vi "assignment_cont.vi"() -> ()   [LabVIEW 2014]
uses:
  <vilib>/DAQmx/create/channels.llb/DAQmx Create Channel (AI-Voltage-Basic).vi
  <vilib>/DAQmx/read.llb/DAQmx Read (Analog 1D DBL NChan 1Samp).vi
  <vilib>/Utility/file.llb/Write To Spreadsheet File (string).vi
  <vilib>/Utility/file.llb/Write To Spreadsheet File (DBL).vi
panel:
  out "elapsed time(sec)":dbl
  out "XY Graph":cluster{dbl[], dbl[]}[](graph)
  in  "while loop delay time in sec":dbl
  in  "stop":bool
  in  "physical input channels":tag
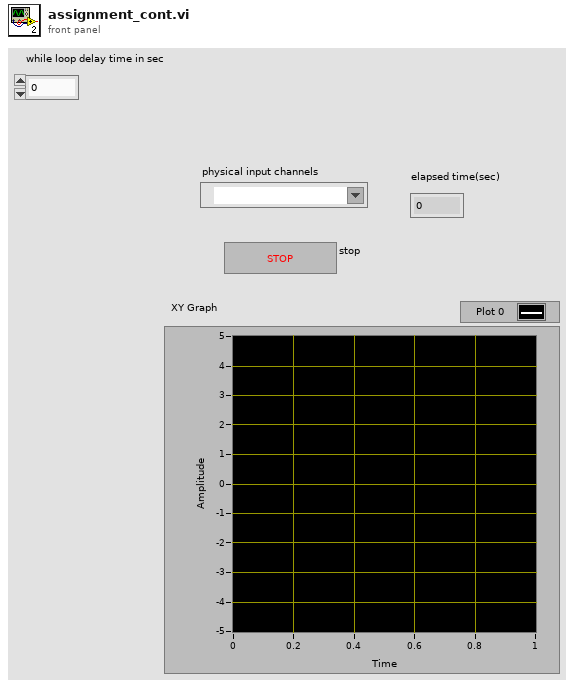
[diagram p1: front panel]
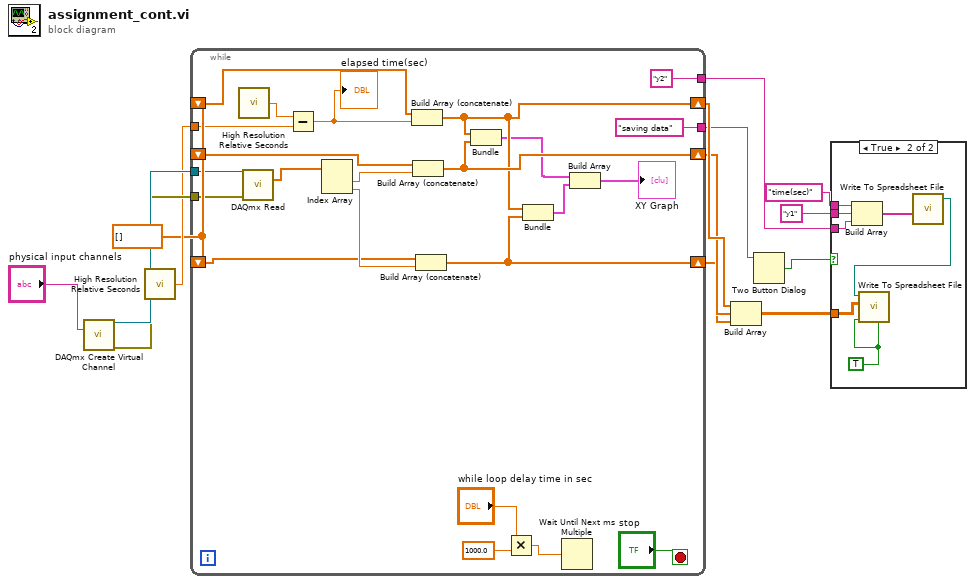
[diagram p0: block diagram]
diagram:
  w10 = dbl[] []
  n1 = call-poly <vilib>:"DAQmx Create Virtual Channel.vi"("physical channels"="physical input channels") -> ("task out"=w14:refnum<k21>, "error out"=w13:errorcluster)  [unwired: 13 in]
  n2 = call <vilib>:"High Resolution Relative Seconds.vi"() -> ("relative seconds"=w11:dbl)
  n3 = while {
    tunnel: w14 -> [w37]
    tunnel: w13 -> [w36]
    tunnel: w11 -> [w30]
    shift-right: [w22] -> w9
    shift-left: w10 -> [w29]
    shift-right: [w23] -> w8
    shift-left: w10 -> [w26]
    shift-right: [w21] -> w7
    shift-left: w10 -> [w24]
    tunnel: ["y2"] -> w3
    tunnel: ["saving data" ("message")] -> w1
    stop <- "stop" stop-if-true
    n4 = call <vilib>:"High Resolution Relative Seconds.vi"() -> ("relative seconds"=w31:dbl)
    n5 = call-poly <vilib>:"DAQmx Read.vi"("task/channels in"=w37, "error in"=w36) -> ("data"=w28:dbl[])  [unwired: 11 in, 2 out]
    n6 = Subtract(x=w31, y=w30) -> (x-y=w15:dbl)
    "elapsed time(sec)" <- w15
    n7 = Index Array(array=w28) -> (element #1=w27:dbl, element #2=w25:dbl)  [unwired: 2 in]
    n8 = Build Array (concatenate)(w29, w15) -> (w22:dbl[])
    n9 = Build Array (concatenate)(w26, w27) -> (w23:dbl[])
    n10 = Build Array (concatenate)(w24, w25) -> (w21:dbl[])
    n11 = Bundle(w22, w23) -> (w20:cluster{dbl[], dbl[]})  [unwired: 1 in]
    n12 = Multiply(x="while loop delay time in sec", y=1000.0) -> (x*y=w34:dbl)
    n13 = Bundle(w22, w21) -> (w19:cluster{dbl[], dbl[]})  [unwired: 1 in]
    n14 = Wait Until Next ms Multiple(millisecond multiple=w34) -> ()  [unwired: 1 out]
    n15 = Build Array(w20, w19) -> (→"XY Graph":cluster{dbl[], dbl[]}[])
  }
  n16 = Build Array(w9, w8, w7) -> (w6:dbl[][])
  n17 = Two Button Dialog(message=w1) -> (T button?=w2:bool)  [unwired: 2 in]
  n18 = case shown="True" w2 {
    tunnel: w6 -> [_ w44]
    tunnel: "time(sec)" -> [_ w43]
    tunnel: "y1" -> [_ w42]
    tunnel: w3 -> [_ w38]
    frame False {
    }
    frame True {
      w39 = TRUE
      n19 = Build Array(w43, w42, w38) -> (w41:string[])
      n20 = call-poly <vilib>:"Write To Spreadsheet File.vi"("1D data"=w41) -> ("new file path (Not A Path if cancelled)"=w40:path)  [unwired: 7 in]
      n21 = call-poly <vilib>:"Write To Spreadsheet File.vi"("transpose? (no:F)"=w39, "append to file? (new file:F)"=w39, "2D data"=w44, "file path (dialog if empty)"=w40) -> ()  [unwired: 4 in, 1 out]
    }
  }
